vi "SET GMap Control Ref.vi"(8 "Error In":errorcluster, 11 "Map References":T1) -> (0 "Error Out":errorcluster)   [LabVIEW 2014]
uses:
  SubVI/Reference/Controls/Mapping References.ctl
  C:/Robotic Systems/Products/Surveyor/Software/Ground Station/Data/Mapping DLL/GMap.NET.WindowsForms.dll
  Data/Mapping DLL/GMap.NET.WindowsForms.dll
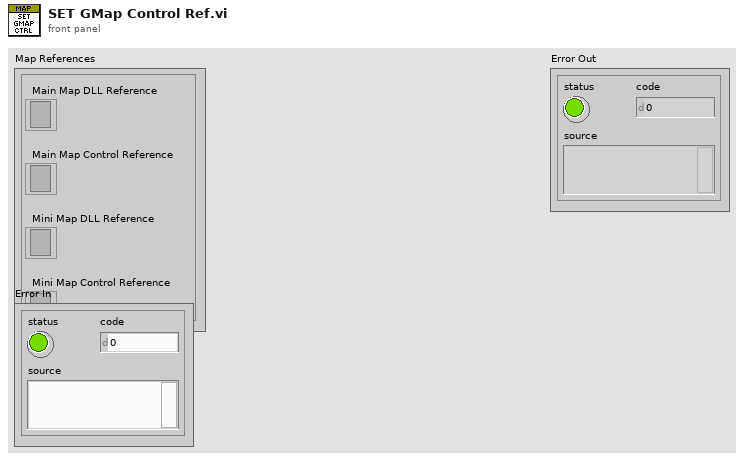
[diagram p1: front panel]
types:
  T1 = typedef "Mapping References.ctl" = cluster{"Main Map DLL Reference":refnum<k24>, "Main Map Control Reference":refnum<k24>, "Mini Map DLL Reference":refnum<k24>, "Mini Map Control Reference":refnum<k24>}
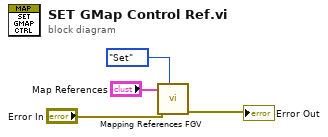
[diagram p0: block diagram]
diagram:
  n1 = call "Mapping References FGV.vi"("Method"=enum16{"Get", "Set"}."Set", "Error In"="Error In", "Map References"="Map References") -> ("Error Out"=→"Error Out":errorcluster)  [unwired: 7 in, 1 out]
